vi "Publish Endpoint.vi"(8 "error in (no error)":errorcluster, 11 "Group in":refnum<class "Group.lvclass">) -> (0 "error out":errorcluster, 2 "Publish Endpoint":T1, 3 "Group out":refnum<class "Group.lvclass">)   [LabVIEW 2020, in "VolatusConfig.lvlib" / "Group.lvclass"]
uses:
  Group.lvclass
  Group.lvclass/Group.ctl
  lv-cdm/CDM-Config/Config Element/Config Element.lvclass
  Endpoint.ctl
  VolatusConfig.lvlib
  VolatusConfigElement/VolatusConfigElement.lvclass
  C:/dev/lv20CE/relink/lv-volatus/VolatusConfig/VolatusConfigElement/VolatusConfigElement.lvclass
  C:/dev/lv20CE/relink/lv-volatus/VolatusConfig/Group/Group.lvclass
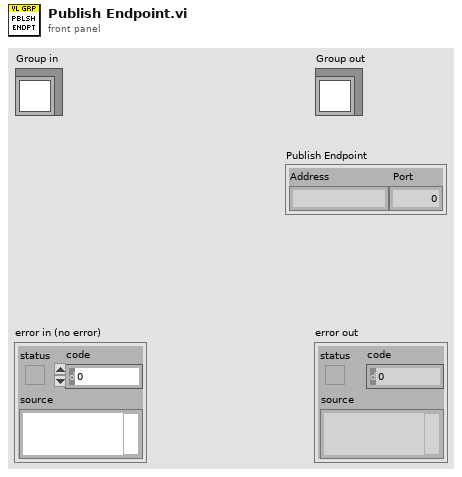
[diagram p1: front panel]
types:
  T1 = typedef "VolatusConfig.lvlib/Endpoint.ctl" = cluster{"Address":string, "Port":u16}
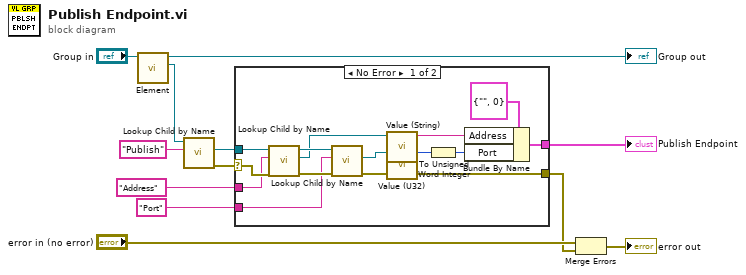
[diagram p0: block diagram]
diagram:
  n1 = call "Element.vi"("VolatusConfigElement in"="Group in") -> ("Element"=w1:refnum<class "Config Element.lvclass">, "VolatusConfigElement out"=→"Group out":refnum<class "Group.lvclass">)  [unwired: 9 in]
  n2 = call "Lookup Child by Name.vi"("Name"="Publish", "Config Element in"=w1) -> ("error out"=w8:errorcluster, "Child"=w9:refnum<class "Config Element.lvclass">)  [unwired: 6 in, 2 out]
  n3 = case shown="No Error" w8 {
    selector: w8 -> [w24 _]
    tunnel: w9 -> [w25 _]
    tunnel: "Address" ("Name") -> [w23 _]
    tunnel: "Port" ("Name") -> [w21 _]
    tunnel: [w14 _] -> w4
    tunnel: [w13 _] -> w3
    frame No Error {
      n4 = call "Lookup Child by Name.vi"("error in (no error)"=w24, "Name"=w23, "Config Element in"=w25) -> ("error out"=w26:errorcluster, "Child"=w15:refnum<class "Config Element.lvclass">, "Config Element out"=w22:refnum<class "Config Element.lvclass">)  [unwired: 5 in, 1 out]
      n5 = call "Lookup Child by Name.vi"("error in (no error)"=w26, "Name"=w21, "Config Element in"=w22) -> ("error out"=w14:errorcluster, "Child"=w19:refnum<class "Config Element.lvclass">)  [unwired: 5 in, 2 out]
      n6 = call "Value (String).vi"("Config Element in"=w15) -> ("String Value"=w16:string)  [unwired: 9 in, 1 out]
      n7 = call "Value (U32).vi"("Config Element in"=w19) -> ("U32 Value"=w18:u32)  [unwired: 9 in, 1 out]
      n8 = To Unsigned Word Integer(number=w18) -> (unsigned 16bit integer=w17:u16)
      n9 = Bundle By Name(cluster=T1 {"Address"="", "Port"=0} ("Endpoint"), "Address"=w16, "Port"=w17) -> (w13:T1)
    }
    frame Error {
      # "Doesn't have publish config which is fine, it just won't be published."
    }
  }
  "Publish Endpoint" <- w3
  n10 = Merge Errors("error in (no error)", w4) -> (→"error out":errorcluster)
